vi "CreateToolbarObject.vi"(0 "reference in":refnum<class "StateDiagramGraph.lvclass">, 2 "GraphButton":u32, 5 "error in (no error)":errorcluster) -> (14 "reference out":refnum<class "StateDiagramGraph.lvclass">, 15 "toolType":T1, 16 "Edge":refnum<class "AbstractEdge.lvclass">, 17 "Node":refnum<class "AbstractNode.lvclass">, 18 "ButtonNameCompressed)":string, 19 "error out":errorcluster)   [LabVIEW 2016, in "StateDiagramGraph.lvclass"]
uses:
  <resource>/Framework/Providers/Open_GDS/UML/StateDiagramGraph_class/StateDiagramGraph.lvclass
  <resource>/Framework/Providers/Open_GDS/UML/UMLEditor/UMLEditor tooltype.ctl
  <resource>/Framework/Providers/Open_GDS/UML/AbstractEdge_class/AbstractEdge.lvclass
  <resource>/Framework/Providers/Open_GDS/UML/AbstractNode_class/AbstractNode.lvclass
  <resource>/Framework/Providers/Open_GDS/UML/ArrowHead_class/ArrowHeadType.ctl
  <resource>/Framework/Providers/Open_GDS/UML/BentStyle_class/BentStyleType.ctl
  <resource>/Framework/Providers/Open_GDS/UML/LineStyle_class/LineStyleType.ctl
  <resource>/Framework/Providers/Open_GDS/UML/Graph_class/ToolbarButtonType.ctl
  <resource>/Framework/Providers/Open_GDS/UML/StateNode_class/StateNode.lvclass
  C:/Program Files (x86)/National Instruments/LabVIEW 2016/resource/Framework/Providers/Open_GDS/UML/RectangularNode_class/RectangularNode.lvclass
  <resource>/Framework/Providers/Open_GDS/UML/InitialStateNode_class/InitialStateNode.lvclass
  <resource>/Framework/Providers/Open_GDS/UML/FinalStateNode_class/FinalStateNode.lvclass
  <resource>/Framework/Providers/Open_GDS/UML/NoteNode_class/NoteNode.lvclass
  <resource>/Framework/Providers/Open_GDS/UML/ChoiceNode_class/ChoiceNode.lvclass
  <resource>/Framework/Providers/Open_GDS/UML/StateTransitionEdge_class/StateTransitionEdge.lvclass
  C:/Program Files (x86)/National Instruments/LabVIEW 2016/resource/Framework/Providers/Open_GDS/UML/GeneralPathEdge_class/GeneralPathEdge.lvclass
  <resource>/Framework/Providers/Open_GDS/UML/NoteEdge_class/NoteEdge.lvclass
  <resource>/Framework/Providers/Open_GDS/UML/GeneralPathEdge_class/GeneralPathEdge.lvclass
  C:/Program Files (x86)/National Instruments/LabVIEW 2016/resource/Framework/Providers/Open_GDS/UML/AbstractEdge_class/AbstractEdge.lvclass
  <resource>/Framework/Providers/Open_GDS/UML/RectangularNode_class/RectangularNode.lvclass
  C:/Program Files (x86)/National Instruments/LabVIEW 2016/resource/Framework/Providers/Open_GDS/UML/AbstractNode_class/AbstractNode.lvclass
  <resource>/Framework/Providers/Open_GDS/UML/ArrowHead_class/ArrowHead.lvclass
  <resource>/Framework/Providers/Open_GDS/UML/BentStyle_class/BentStyle.lvclass
  <resource>/Framework/Providers/Open_GDS/UML/LineStyle_class/LineStyle.lvclass
  <resource>/Framework/Providers/Open_GDS/UML/Graph_class/Graph.lvclass
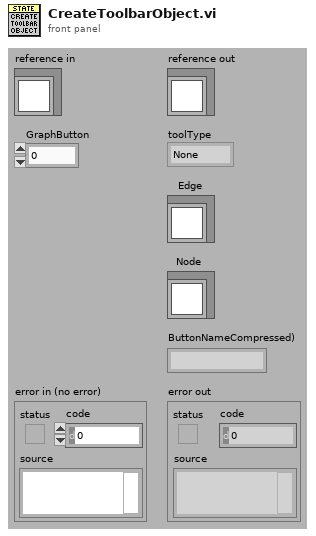
[diagram p1: front panel]
types:
  T1 = typedef "UMLEditor tooltype.ctl" = enum16{"None", "Node", "Edge"}
  T2 = typedef "Graph.lvclass/ToolbarButtonType.ctl" = cluster{"Text":string, "Type":T1}
  T3 = typedef "LineStyle.lvclass/LineStyleType.ctl" = enum16{"SOLID", "DOTTED"}
  T4 = typedef "BentStyle.lvclass/BentStyleType.ctl" = enum16{"STRAIGHT", "HV", "VH", "HVH", "VHV", "ARC"}
  T5 = typedef "ArrowHead.lvclass/ArrowHeadType.ctl" = enum16{"NONE", "TRIANGLE", "BLACK_TRIANGLE", "V", "HALF_V", "DIAMOND", "BLACK_DIAMOND"}
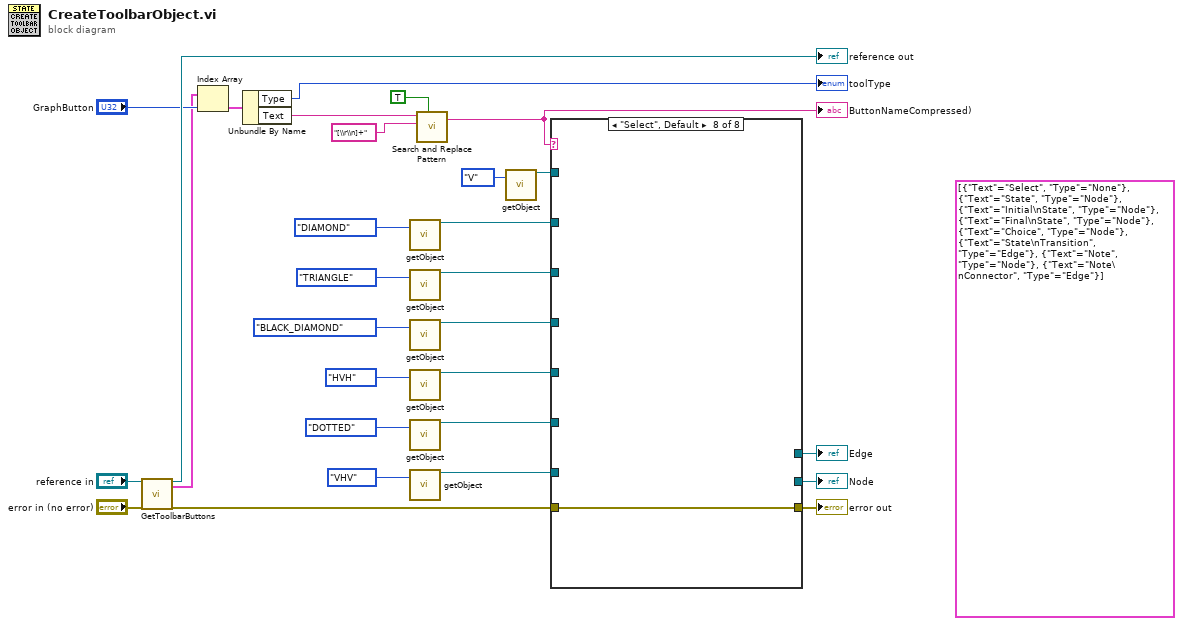
[diagram p0: block diagram]
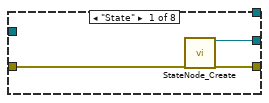
[diagram p2: hidden frame]
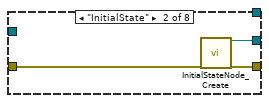
[diagram p3: hidden frame]
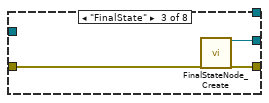
[diagram p4: hidden frame]
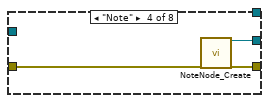
[diagram p5: hidden frame]
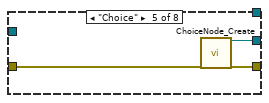
[diagram p6: hidden frame]
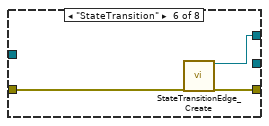
[diagram p7: hidden frame]
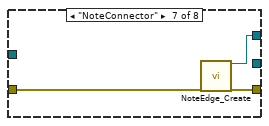
[diagram p8: hidden frame]
diagram:
  (unwired) T2[] [{"Text"="Select", "Type"=enum."None"}, {"Text"="State", "Type"=enum."Node"}, {"Text"="Initial\nState", "Type"=enum."Node"}, {"Text"="Final\nState", "Type"=enum."Node"}, {"Text"="Choice", "Type"=enum."Node"}, {"Text"="State\nTransition", "Type"=enum."Edge"}, {"Text"="Note", "Type"=enum."Node"}, {"Text"="Note\nConnector", "Type"=enum."Edge"}] ("ToolbarButtons")
  n1 = call-dynamic "GetToolbarButtons.vi"("reference in"="reference in", "error in (no error)"="error in (no error)") -> ("reference out"=→"reference out":refnum<class "StateDiagramGraph.lvclass">, "ToolbarButtons"=w20:T2[], "error out"=w11:errorcluster)  [unwired: 13 in, 2 out]
  n2 = Index Array(array=w20, index="GraphButton") -> (element=w19:T2)
  n3 = Unbundle By Name(w19) -> ("Type"=→"toolType":T1, "Text"=w3:string)
  n4 = call <resource>:"getObject.vi"("arrowHead"=ArrowHeadType."DIAMOND") -> ("reference out"=w5:refnum<class "ArrowHead.lvclass">)  [unwired: 1 in, 17 out]
  n5 = call <resource>:"getObject.vi"("arrowHead"=ArrowHeadType."TRIANGLE") -> ("reference out"=w7:refnum<class "ArrowHead.lvclass">)  [unwired: 1 in, 17 out]
  n6 = call <resource>:"getObject.vi"("arrowHead"=ArrowHeadType."BLACK_DIAMOND") -> ("reference out"=w4:refnum<class "ArrowHead.lvclass">)  [unwired: 1 in, 17 out]
  n7 = call <resource>:"getObject.vi"("bentStyle"=BentStyleType."HVH") -> ("reference out"=w6:refnum<class "BentStyle.lvclass">)  [unwired: 1 in, 17 out]
  n8 = call <resource>:"getObject.vi"("lineStyle"=LineStyleType."DOTTED") -> ("reference out"=w10:refnum<class "LineStyle.lvclass">)  [unwired: 1 in, 17 out]
  n9 = call <resource>:"getObject.vi"("bentStyle"=BentStyleType."VHV") -> ("reference out"=w8:refnum<class "BentStyle.lvclass">)  [unwired: 1 in, 17 out]
  n10 = call <vilib>:"Search and Replace Pattern.vi"("string"=w3, "regular expression (\"\")"="[\\r\\n]+" ("regular expression (\"\")"), "replace all? (F)"=TRUE) -> ("result string"=w21:string)  [unwired: 2 in, 1 out]
  "ButtonNameCompressed)" <- w21
  n11 = call <resource>:"getObject.vi"("arrowHead"=ArrowHeadType."V") -> ("reference out"=w9:refnum<class "ArrowHead.lvclass">)  [unwired: 1 in, 17 out]
  n12 = case shown="\"Select\", Default" w21 {
    tunnel: w11 -> [w32 w35 w36 w41 w44 w47 w50 w51]
    tunnel: [w31 w34 w38 w40 w43 w46 w49 w51] -> w28
    tunnel: [w30 w33 w37 w39 w42 _ _ _] -> w23
    tunnel: w10 -> [_ _ _ _ _ _ _ _]
    tunnel: w9 -> [_ _ _ _ _ _ _ _]
    tunnel: w8 -> [_ _ _ _ _ _ _ _]
    tunnel: w7 -> [_ _ _ _ _ _ _ _]
    tunnel: w6 -> [_ _ _ _ _ _ _ _]
    tunnel: w5 -> [_ _ _ _ _ _ _ _]
    tunnel: w4 -> [_ _ _ _ _ _ _ _]
    tunnel: [_ _ _ _ _ w45 w48 _] -> w22
    frame "State" {
      n13 = call <resource>:"StateNode_Create.vi"("error in (no error)"=w32) -> ("reference out"=w30:refnum<class "StateNode.lvclass">, "error out"=w31:errorcluster)  [unwired: 17 in]
    }
    frame "InitialState" {
      n14 = call <resource>:"InitialStateNode_Create.vi"("error in (no error)"=w35) -> ("reference out"=w33:refnum<class "InitialStateNode.lvclass">, "error out"=w34:errorcluster)  [unwired: 17 in]
    }
    frame "FinalState" {
      n15 = call <resource>:"FinalStateNode_Create.vi"("error in (no error)"=w36) -> ("reference out"=w37:refnum<class "FinalStateNode.lvclass">, "error out"=w38:errorcluster)  [unwired: 17 in]
    }
    frame "Note" {
      n16 = call <resource>:"NoteNode_Create.vi"("error in (no error)"=w41) -> ("reference out"=w39:refnum<class "NoteNode.lvclass">, "error out"=w40:errorcluster)  [unwired: 1 in, 16 out]
    }
    frame "Choice" {
      n17 = call <resource>:"ChoiceNode_Create.vi"("error in (no error)"=w44) -> ("reference out"=w42:refnum<class "ChoiceNode.lvclass">, "error out"=w43:errorcluster)  [unwired: 17 in]
    }
    frame "StateTransition" {
      n18 = call <resource>:"StateTransitionEdge_Create.vi"("error in (no error)"=w47) -> ("reference out"=w45:refnum<class "StateTransitionEdge.lvclass">, "error out"=w46:errorcluster)  [unwired: 1 in, 16 out]
    }
    frame "NoteConnector" {
      n19 = call <resource>:"NoteEdge_Create.vi"("error in (no error)"=w50) -> ("reference out"=w48:refnum<class "NoteEdge.lvclass">, "error out"=w49:errorcluster)  [unwired: 1 in, 16 out]
    }
    frame "Select", Default {
    }
  }
  "error out" <- w28
  "Edge" <- w22
  "Node" <- w23
